vi "Side Horizontal.vi"(0 "Image In":T2(plugin-control), 1 "Ref ROI Descriptor":T1 {"Contours"."Type" items=["No Selection", "Point", "Line", "Rectangle", "Oval", "Polygon", "Free", "Annulus", "Unused2", "Unused3", "Broken Line", "Free Hand Line", "Rotated Rectangle"]}, 2 "ROI 1":T8 {"Contours"."Type" items=["No Selection", "Point", "Line", "Rectangle", "Oval", "Polygon", "Freehand Region", "Annulus", "Unused2", "Unused3", "Broken Line", "Freehand Line", "Rotated Rectangle"]}, 3 "Edge Options Ref ROI":T4={"Edge Polarity"=2, "Kernel Size"=5, "Width"=5, "Minimum Edge Strength"=50.0, "Interpolation Type"=enum."Bilinear Fixed", "Data Processing Method"=enum."Average"} {"Edge Polarity" items=["All Edges", "Rising Edges", "Falling Edges"]; "Minimum Edge Strength" format="%.2f"; "Width" step=2; "Kernel Size" step=2}, 4 "Edge Options ROI 1":T4={"Edge Polarity"=0, "Kernel Size"=5, "Width"=5, "Minimum Edge Strength"=50.0, "Interpolation Type"=enum."Bilinear Fixed", "Data Processing Method"=enum."Average"} {"Edge Polarity" items=["All Edges", "Rising Edges", "Falling Edges"]; "Minimum Edge Strength" format="%.2f"; "Width" step=2; "Kernel Size" step=2}, 5 "Ref ROI Search Direction":u32(ring)=2 items=["Left to Right", "Right to Left", "Top to Bottom", "Bottom to Top"], 6 "Search Direction ROI 1":u32(ring) items=["Left to Right", "Right to Left", "Top to Bottom", "Bottom to Top"], 7 "error in (no error)":errorcluster, 8 "Calib Image":T2, 9 "Line Options Ref ROI":T6={"Number of Lines"=1, "Type"=enum."First Edge Rake", "Min. Score"=10.0, "Max. Score"=1000.0, "Orientation"=10.0, "Angle Range"=60.0, "Angle Tolerance"=10.0, "Step Size"=6, "Min. SNR (db)"=0.0, "Min. Points (%)"=25.0, "Hough Iterations"=5} {"Min. Points (%)" min=0.0 max=100.0; "Min. SNR (db)" min=0.0; "Max. Score" min=0.0 max=1024.0; "Min. Score" min=0.0 max=1024.0 step=1.0}, 10 "Step Size ROI 1":u32=3, 11 "Process ROI 1":T3(ring)=enum."Get First + Last Edge", 12 "Overlay ROI":bool, 13 "Overlay Rake Lines":bool, 14 "Overlay Points":bool) -> (20 "First Overlay Line":T10, 21 "Second Overlay Line":T9, 22 "Mesurement Value":sgl, 27 "error out":errorcluster)   [LabVIEW 2019, in "Algorithm.lvclass"]
uses:
  FrameworkOverrides/Algorithm.lvclass
  <vilib>/vision/NI_Vision_Development_Module.lvlib
  <vilib>/vision/Measure.llb/Edge New.ctl
  <vilib>/vision/Measure.llb/Edge Polarity.ctl
  <vilib>/vision/Measure.llb/Edge Options.ctl
  <vilib>/vision/Measure.llb/Straight Edge Process.ctl
  <vilib>/vision/Measure.llb/Straight Edge Options.ctl
  <vilib>/vision/Image Controls.llb/IMAQ Image.ctl
panel:
  in  "AvgMinMax":enum16{"Average", "Max", "Min", "Max2"}(ring)
  out "Last Edges":T11[](array[typedef]) {"Distance (Real-World)" format="%.2f"; "Location (Real-World)"."Y" format="%.2g"; "Location (Real-World)"."X" format="%.2f"; "Noise" format="%.2f"; "Location (Pixel)"."Y" format="%.2g"; "Location (Pixel)"."X" format="%.2f"; "Strength" format="%.2f"; "Distance (Pixel)" format="%.2f"}
  out "First Edges":T11[](array[typedef]) {"Distance (Real-World)" format="%.2f"; "Location (Real-World)"."Y" format="%.2g"; "Location (Real-World)"."X" format="%.2f"; "Noise" format="%.2f"; "Location (Pixel)"."Y" format="%.2g"; "Location (Pixel)"."X" format="%.2f"; "Strength" format="%.2f"; "Distance (Pixel)" format="%.2f"}
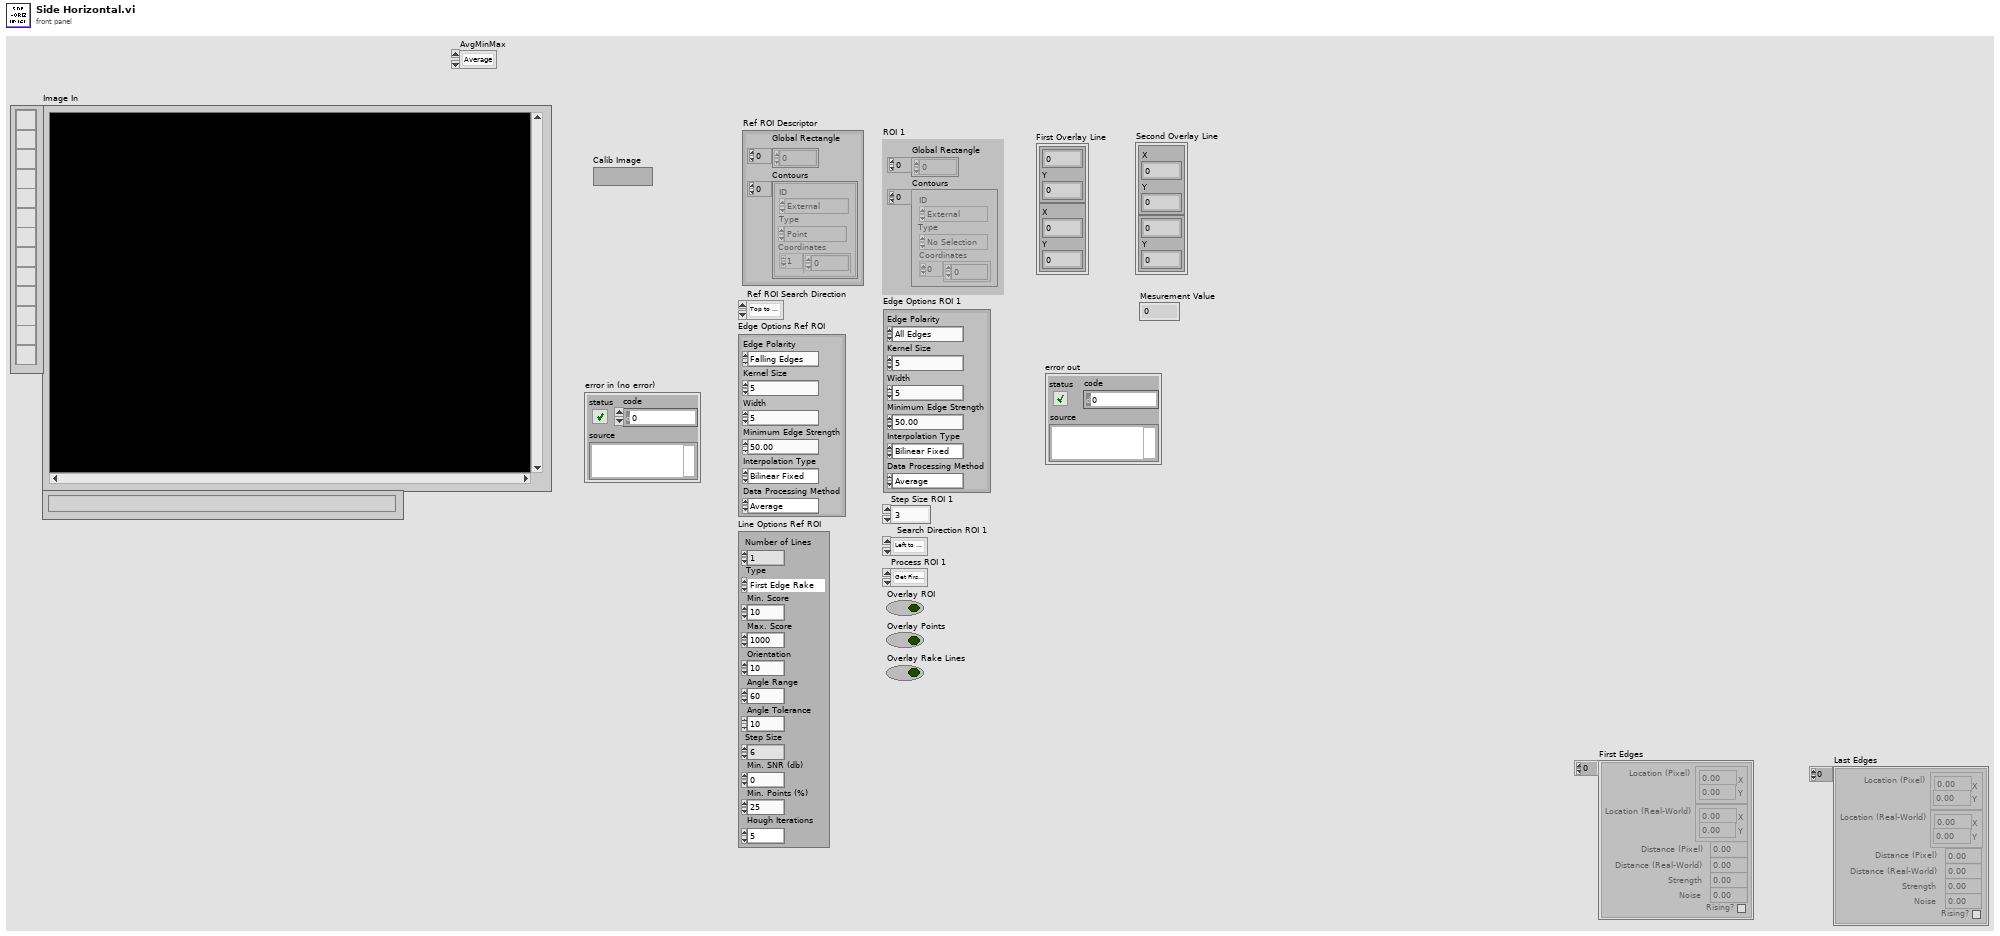
[diagram p1: front panel]
types:
  T1 = cluster{"Global Rectangle":i32[], "Contours":cluster{"ID":enum32{"External", "Internal"}, "Type":u32, "Coordinates":i32[]}[]}
  T2 = typedef "IMAQ Image.ctl" = refnum<image>
  T3 = enum16{"Get First Edge", "Get First + Last Edge", "Get All Edges", "Get Best Edge"}
  T4 = typedef "Edge Options.ctl" = cluster{"Edge Polarity":T5, "Kernel Size":u32, "Width":u32, "Minimum Edge Strength":sgl, "Interpolation Type":enum32{"Zero Order", "Bilinear", "Quadratic", "Cubic", "Bilinear Fixed"}, "Data Processing Method":enum32{"Average", "Median"}}
  T5 = typedef "Edge Polarity.ctl" = u32
  T6 = typedef "Straight Edge Options.ctl" = cluster{"Number of Lines":i32, "Type":T7, "Min. Score":dbl, "Max. Score":dbl, "Orientation":dbl, "Angle Range":dbl, "Angle Tolerance":dbl, "Step Size":u32, "Min. SNR (db)":dbl, "Min. Points (%)":dbl, "Hough Iterations":i32}
  T7 = typedef "Straight Edge Process.ctl" = enum32{"First Edge Rake", "Best Edge Rake", "Hough Edge Rake", "First Edge Projection", "Best Edge Projection"}
  T8 = typedef "ROI Descriptor" = cluster{"Global Rectangle":i32[], "Contours":cluster{"ID":enum32{"External", "Internal"}, "Type":u32, "Coordinates":i32[]}[]}
  T9 = cluster{cluster{"X":sgl, "Y":sgl}, cluster{sgl, "Y":sgl}}
  T10 = cluster{cluster{sgl, "Y":sgl}, cluster{"X":sgl, "Y":sgl}}
  T11 = typedef "Edge New.ctl" = cluster{"Location (Pixel)":cluster{"X":sgl, "Y":sgl}, "Location (Real-World)":cluster{"X":sgl, "Y":sgl}, "Distance (Pixel)":dbl, "Distance (Real-World)":dbl, "Strength":dbl, "Noise":dbl, "Rising?":bool}
  T12 = cluster{"Contrast":i32, "Filter width":i32, "Steepness":i32, "Subsampling Ratio":u32, "Show Search Area":bool, "Show Search Lines":bool, "Show Edges Found":bool, "Show Result":bool}
  T13 = typedef "IMAQ Rectangle" = cluster{"Left":i32, "Top":i32, "Right":i32, "Bottom":i32, "Rotation":dbl}
  T14 = cluster{"Point1 (Pixels)":cluster{"X":sgl, "Y":sgl}, "Point2 (Pixels)":cluster{"X":sgl, "Y":sgl}, "Point1 (Real-World)":cluster{"X":sgl, "Y":sgl}, "Point2 (Real-World)":cluster{"X":sgl, "Y":sgl}, "Angle (Pixel)":dbl, "Angle (Real-World)":dbl, "Score":dbl, "Straightness":dbl, "Average SNR (db)":dbl, "Calibration Valid":bool}[]
  T15 = typedef "Search Line.ctl" = cluster{"Start Point":cluster{"X":sgl, "Y":sgl}, "End Point":cluster{"X":sgl, "Y":sgl}, "Edge Info":T11[], "Edge Map":dbl[], "Calibration Valid":bool}
  T16 = cluster{"Point1 (Pixels)":cluster{"X":sgl, "Y":sgl}, "Point2 (Pixels)":cluster{"X":sgl, "Y":sgl}, "Point1 (Real-World)":cluster{"X":sgl, "Y":sgl}, "Point2 (Real-World)":cluster{"X":sgl, "Y":sgl}, "Angle (Pixel)":dbl, "Angle (Real-World)":dbl, "Score":dbl, "Straightness":dbl, "Average SNR (db)":dbl, "Calibration Valid":bool}
  T17 = cluster{"Location (Pixel)":cluster{"X":sgl, "Y":sgl}, "Location (Pixel)":cluster{"X":sgl, "Y":sgl}}
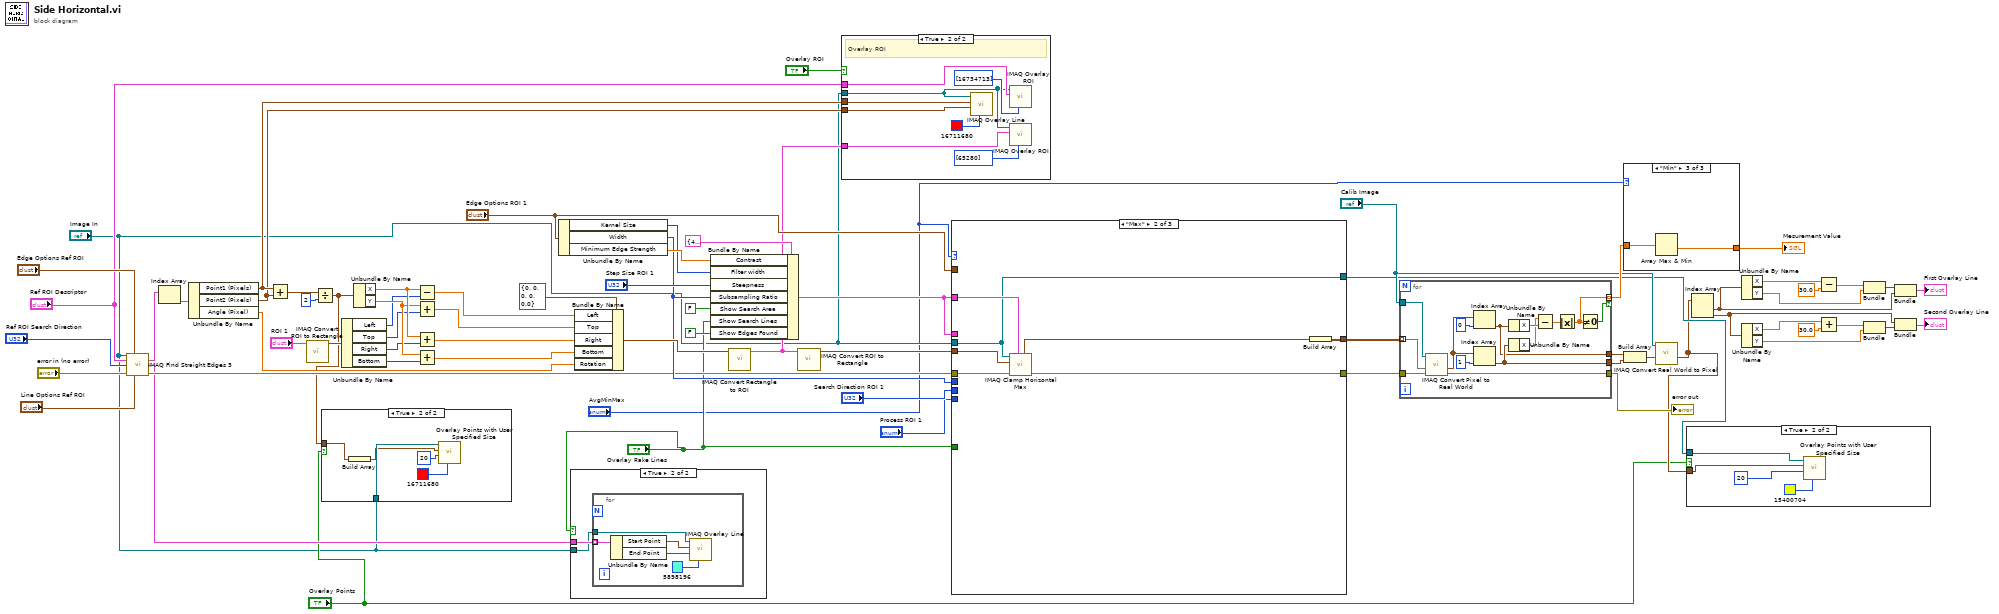
[diagram p0: block diagram]
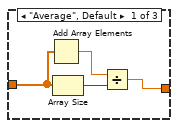
[diagram p6: hidden frame]
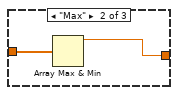
[diagram p7: hidden frame]
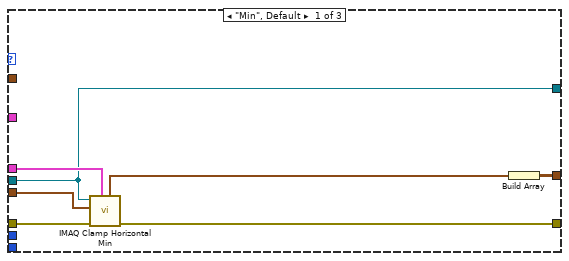
[diagram p8: hidden frame]
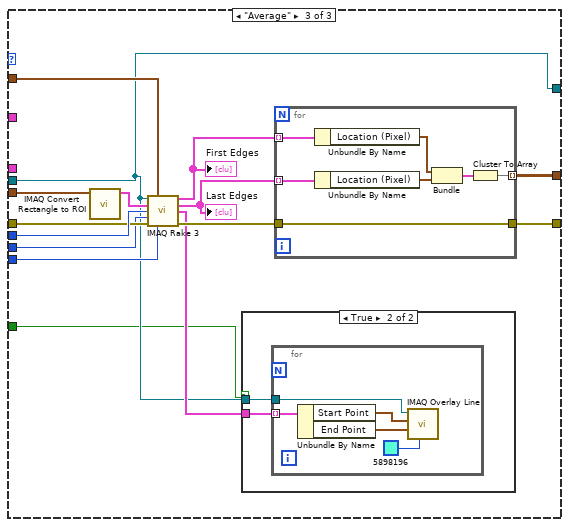
[diagram p9: hidden frame]
diagram:
  n1 = call "IMAQ Find Straight Edges 3"("Image"="Image In", "Edge Options"="Edge Options Ref ROI", "ROI Descriptor"="Ref ROI Descriptor", "Search Direction"="Ref ROI Search Direction", "error in (no error)"="error in (no error)", "Line Options"="Line Options Ref ROI") -> ("Straight Edges"=w69:T14, "Search Lines Information"=w5:T15[], "error out"=w48:errorcluster)  [unwired: 5 in, 2 out]
  n2 = Index Array(array=w69) -> (element=w68:T16)  [unwired: 1 in]
  n3 = Unbundle By Name(w68) -> ("Point1 (Pixels)"=w12:cluster{"X":sgl, "Y":sgl}, "Point2 (Pixels)"=w11:cluster{"X":sgl, "Y":sgl}, "Angle (Pixel)"=w58:dbl)
  n4 = Add(x=w12, y=w11) -> (x+y=w67:cluster{"X":sgl, "Y":sgl})
  n5 = call "IMAQ Convert ROI to Rectangle"("ROI Descriptor"="ROI 1") -> ("Rectangle"=w23:T13)  [unwired: 8 in, 1 out]
  n6 = Divide(x=w67, y=2) -> (x/y=w3:cluster{"X":sgl, "Y":sgl})
  n7 = case shown="True" "Overlay Points" {
    tunnel: w3 -> [_ w74]
    tunnel: "Image In" -> [_ w75]
    frame False {
    }
    frame True {
      n8 = Build Array(w74) -> (w73:cluster{"X":sgl, "Y":sgl}[])
      n9 = call "Overlay Points with User Specified Size.vi"("Color"=u32 16711680, "Point Diameter (5)"=u32 20, "Points"=w73, "Image In"=w75) -> ()  [unwired: 6 in, 2 out]
    }
  }
  n10 = Unbundle By Name(w23) -> ("Left"=w22:i32, "Top"=w20:i32, "Right"=w21:i32, "Bottom"=w19:i32)
  n11 = Unbundle By Name(w3) -> ("X"=w65:sgl, "Y"=w61:sgl)
  n12 = Subtract(x=w65, y=w22) -> (x-y=w63:sgl)
  n13 = Add(x=w61, y=w20) -> (x+y=w60:sgl)
  n14 = Add(x=w65, y=w21) -> (x+y=w62:sgl)
  n15 = Add(x=w61, y=w19) -> (x+y=w59:sgl)
  n16 = Unbundle By Name("Edge Options ROI 1") -> ("Kernel Size"=w53:u32, "Width"=w52:u32, "Minimum Edge Strength"=w54:sgl)
  n17 = case shown="True" "Overlay Rake Lines" {
    tunnel: w5 -> [_ w79]
    tunnel: "Image In" -> [_ w78]
    frame False {
    }
    frame True {
      n18 = for {
        tunnel: w79 -> [w84] mode=indexing
        tunnel: w78 -> [w83]
        n19 = Unbundle By Name(w84) -> ("Start Point"=w82:cluster{"X":sgl, "Y":sgl}, "End Point"=w81:cluster{"X":sgl, "Y":sgl})
        n20 = call "IMAQ Overlay Line"("Color"=u32 5898196, "End Point"=w81, "Start Point"=w82, "Image"=w83) -> ()  [unwired: 6 in, 2 out]
      }
    }
  }
  n21 = Bundle By Name(cluster=T13 {"Left"=0, "Top"=0, "Right"=0, "Bottom"=0, "Rotation"=0.0} ("Rectangle"), "Left"=w63, "Top"=w60, "Right"=w62, "Bottom"=w59, "Rotation"=w58) -> (w57:T13)
  n22 = Bundle By Name(cluster=T12 {"Contrast"=40, "Filter width"=4, "Steepness"=2, "Subsampling Ratio"=5, "Show Search Area"=FALSE, "Show Search Lines"=FALSE, "Show Edges Found"=FALSE, "Show Result"=TRUE} ("Settings"), "Contrast"=w54, "Filter width"=w53, "Steepness"=w52, "Subsampling Ratio"="Step Size ROI 1", "Show Search Area"=FALSE, "Show Search Lines"="Overlay Rake Lines", "Show Edges Found"=FALSE) -> (w51:T12)
  n23 = call "IMAQ Convert Rectangle to ROI"("Rectangle"=w57) -> ("ROI Descriptor"=w10:T8)  [unwired: 8 in, 1 out]
  n24 = call "IMAQ Convert ROI to Rectangle"("ROI Descriptor"=w10) -> ("Rectangle"=w56:T13)  [unwired: 8 in, 1 out]
  n25 = case shown="True" "Overlay ROI" {
    tunnel: "Ref ROI Descriptor" -> [_ w92]
    tunnel: "Image In" -> [_ w86]
    tunnel: w12 -> [_ w90]
    tunnel: w11 -> [_ w89]
    tunnel: w10 -> [_ w87]
    frame False {
    }
    frame True {
      # "Overlay ROI"
      n26 = call "IMAQ Overlay Line"("Color"=u32 16711680, "End Point"=w89, "Start Point"=w90, "Image"=w86) -> ()  [unwired: 6 in, 2 out]
      n27 = call "IMAQ Overlay ROI"("Colors (Green)"=u32[] [16734713], "ROI Descriptor"=w92, "Image"=w86) -> ()  [unwired: 7 in, 2 out]
      n28 = call "IMAQ Overlay ROI"("Colors (Green)"=u32[] [65280], "ROI Descriptor"=w87, "Image"=w86) -> ()  [unwired: 7 in, 2 out]
    }
  }
  n29 = case shown="\"Max\"" "AvgMinMax" {
    tunnel: w56 -> [w99 w106 w121]
    tunnel: "Image In" -> [w96 w102 w108]
    tunnel: [w93 w100 w113] -> w43
    tunnel: w51 -> [w98 _ _]
    tunnel: w51 -> [_ w105 _]
    tunnel: "Edge Options ROI 1" -> [_ _ w117]
    tunnel: "Step Size ROI 1" -> [_ _ w115]
    tunnel: w48 -> [w95 w104 w114]
    tunnel: [w97 w103 w112] -> w42
    tunnel: [w96 w102 w108] -> w8
    tunnel: "Search Direction ROI 1" -> [_ _ w111]
    tunnel: "Process ROI 1" -> [_ _ w110]
    tunnel: "Overlay Rake Lines" -> [_ _ w107]
    frame "Min", Default {
      n30 = call "IMAQ Clamp Horizontal Min"("Settings"=w98, "error in (no error)"=w95, "Rectangle"=w99, "Image"=w96) -> ("error out"=w97:errorcluster, "Edge Coordinates"=w94:cluster{"X":sgl, "Y":sgl}[])  [unwired: 3 in, 3 out]
      n31 = Build Array(w94) -> (w93:cluster{"X":sgl, "Y":sgl}[][])
    }
    frame "Max" {
      n32 = call "IMAQ Clamp Horizontal Max"("Settings"=w105, "error in (no error)"=w104, "Rectangle"=w106, "Image"=w102) -> ("error out"=w103:errorcluster, "Edge Coordinates"=w101:cluster{"X":sgl, "Y":sgl}[])  [unwired: 3 in, 3 out]
      n33 = Build Array(w101) -> (w100:cluster{"X":sgl, "Y":sgl}[][])
    }
    frame "Average" {
      n34 = call "IMAQ Convert Rectangle to ROI"("Rectangle"=w121) -> ("ROI Descriptor"=w116:T8)  [unwired: 8 in, 1 out]
      n35 = call "IMAQ Rake 3"("Image"=w108, "Edge Options"=w117, "ROI Descriptor"=w116, "Step Size"=w115, "Scan Direction"=w111, "error in (no error)"=w114, "Process"=w110) -> ("First Edges"=w119:T11[], "Last Edges"=w120:T11[], "Search Lines"=w109:T15[], "error out"=w118:errorcluster)  [unwired: 5 in]
      "First Edges" <- w119
      "Last Edges" <- w120
      n36 = case shown="True" w107 {
        tunnel: w109 -> [_ w123]
        tunnel: w108 -> [_ w122]
        frame False {
        }
        frame True {
          n37 = for {
            tunnel: w123 -> [w128] mode=indexing
            tunnel: w122 -> [w127]
            n38 = Unbundle By Name(w128) -> ("Start Point"=w126:cluster{"X":sgl, "Y":sgl}, "End Point"=w125:cluster{"X":sgl, "Y":sgl})
            n39 = call "IMAQ Overlay Line"("Color"=u32 5898196, "End Point"=w125, "Start Point"=w126, "Image"=w127) -> ()  [unwired: 6 in, 2 out]
          }
        }
      }
      n40 = for {
        tunnel: w119 -> [w135] mode=indexing
        tunnel: w120 -> [w134] mode=indexing
        tunnel: w118 -> [w133]
        tunnel: [w133] -> w112
        tunnel: [w129] -> w113 mode=indexing
        n41 = Unbundle By Name(w135) -> ("Location (Pixel)"=w132:cluster{"X":sgl, "Y":sgl})
        n42 = Unbundle By Name(w134) -> ("Location (Pixel)"=w131:cluster{"X":sgl, "Y":sgl})
        n43 = Bundle("Location (Pixel)"=w132, "Location (Pixel)"=w131) -> (w130:T17)  [unwired: 1 in]
        n44 = Cluster To Array(cluster=w130) -> (array=w129:cluster{"X":sgl, "Y":sgl}[])
      }
    }
  }
  n45 = for {
    tunnel: w43 -> [w149] mode=indexing
    tunnel: "Calib Image" -> [w148]
    tunnel: [w143] -> w45 mode=indexing if=w144
    tunnel: w42 -> [w146]
    tunnel: [w145] -> w9
    tunnel: [w137] -> w40
    tunnel: [w136] -> w41
    n46 = call "IMAQ Convert Pixel to Real World"("error in (no error)"=w146, "Array of Pixel Coordinates"=w149, "Calibrated Image"=w148) -> ("error out"=w145:errorcluster, "Array of Real World Coordinates"=w147:cluster{"X":sgl, "Y":sgl}[])  [unwired: 3 in, 4 out]
    n47 = Index Array(array=w147, index=0) -> (element=w136:cluster{"X":sgl, "Y":sgl})
    n48 = Index Array(array=w147, index=1) -> (element=w137:cluster{"X":sgl, "Y":sgl})
    n49 = Unbundle By Name(w136) -> ("X"=w141:sgl)
    n50 = Unbundle By Name(w137) -> ("X"=w140:sgl)
    n51 = Subtract(x=w140, y=w141) -> (x-y=w139:sgl)
    n52 = Absolute Value(x=w139) -> (abs(x)=w143:sgl)
    n53 = Not Equal To 0?(x=w143) -> (x != 0?=w144:bool)
  }
  "error out" <- w9
  n54 = case shown="\"Min\"" "AvgMinMax" {
    tunnel: w45 -> [w153 w155 w157]
    tunnel: [w150 w154 w156] -> w44
    frame "Average", Default {
      n55 = Add Array Elements(numeric array=w153) -> (sum=w152:sgl)
      n56 = Array Size(array=w153) -> (size(s)=w151:i32)
      n57 = Divide(x=w152, y=w151) -> (x/y=w150:sgl)
    }
    frame "Max" {
      n58 = Array Max & Min(array=w155) -> (max value=w154:sgl)  [unwired: 3 out]
    }
    frame "Min" {
      n59 = Array Max & Min(array=w157) -> (min value=w156:sgl)  [unwired: 3 out]
    }
  }
  "Mesurement Value" <- w44
  n60 = Build Array(w41, w40) -> (w39:cluster{"X":sgl, "Y":sgl}[])
  n61 = call "IMAQ Convert Real World to Pixel"("Array of Real World Coordinates"=w39, "Calibrated Image"="Calib Image") -> ("Array of Pixel Coordinates"=w7:cluster{"X":sgl, "Y":sgl}[])  [unwired: 4 in, 5 out]
  n62 = case shown="True" "Overlay Points" {
    tunnel: w8 -> [_ w159]
    tunnel: w7 -> [_ w158]
    frame False {
    }
    frame True {
      n63 = call "Overlay Points with User Specified Size.vi"("Color"=u32 15400704, "Point Diameter (5)"=u32 20, "Points"=w158, "Image In"=w159) -> ()  [unwired: 6 in, 2 out]
    }
  }
  n64 = Index Array(array=w7) -> (element #1=w29:cluster{"X":sgl, "Y":sgl}, element #2=w27:cluster{"X":sgl, "Y":sgl})  [unwired: 2 in]
  n65 = Unbundle By Name(w29) -> ("X"=w38:sgl, "Y"=w33:sgl)
  n66 = Unbundle By Name(w27) -> ("X"=w36:sgl, "Y"=w32:sgl)
  n67 = Subtract(x=w38, y=sgl 30.0) -> (x-y=w34:sgl)
  n68 = Add(x=w36, y=sgl 30.0) -> (x+y=w31:sgl)
  n69 = Bundle(w34, "Y"=w33) -> (w30:cluster{sgl, "Y":sgl})  [unwired: 1 in]
  n70 = Bundle(w31, "Y"=w32) -> (w28:cluster{sgl, "Y":sgl})  [unwired: 1 in]
  n71 = Bundle(w30, w29) -> (→"First Overlay Line":T10)  [unwired: 1 in]
  n72 = Bundle(w27, w28) -> (→"Second Overlay Line":T9)  [unwired: 1 in]
